vi "posctrl-drive-fwd-sim.vi"(11 "Motor Demand":dbl) -> (3 "Drive Speed Ft/Sec":dbl)   [LabVIEW 2019]
uses:
  <vilib>/Rock Robotics/WPI/ThirdParty/JAS_Junk/TrajLib/VI/TimeInterpDouble_New.vi
  <vilib>/Rock Robotics/WPI/ThirdParty/JAS_Junk/TrajLib/VI/TimeInterpDouble_AddSample.vi
  <vilib>/Rock Robotics/WPI/ThirdParty/JAS_Junk/TrajLib/VI/TimeInterpDouble_GetSample.vi
  <vilib>/Rock Robotics/WPI/ThirdParty/JAS_Junk/TrajLib/VI/TimeInterpDouble_SetMaxTime.vi
  <vilib>/Rock Robotics/WPI/ThirdParty/JAS_Junk/TrajLib/Util_GetTime.vi
  <vilib>/Rock Robotics/WPI/ThirdParty/JAS_Junk/TrajLib/LinearFilter_ResetToValue.vi
  <vilib>/Rock Robotics/WPI/ThirdParty/JAS_Junk/TrajLib/LinearFilter_Calculate.vi
  <vilib>/Rock Robotics/WPI/ThirdParty/JAS_Junk/TrajLib/VI/TimeInterpDouble_CleanUp.vi
  <vilib>/Rock Robotics/WPI/ThirdParty/JAS_Junk/TrajLib/MathUtil_Interpolate.vi
  <vilib>/Rock Robotics/WPI/ThirdParty/JAS_Junk/TrajLib/VI/Util_GetTime_U32.vi
  <vilib>/Rock Robotics/WPI/ThirdParty/JAS_Junk/TrajLib/VI/Util_GetTime_U64.vi
  <vilib>/gmath/interp.llb/Search Ordered Table.vi
  <vilib>/Rock Robotics/WPI/ThirdParty/JAS_Junk/TrajLib/LinearFilter_MovingAverage.vi
  <vilib>/Rock Robotics/WPI/ThirdParty/JAS_Junk/TrajLib/LinearFilter_LowPassBW1.vi
  <vilib>/Rock Robotics/WPI/ThirdParty/JAS_Junk/TrajLib/LinearFilter_LowPassBW2.vi
  <vilib>/Rock Robotics/WPI/ThirdParty/JAS_Junk/TrajLib/LinearFilter_HighPassBW1.vi
  <vilib>/Rock Robotics/WPI/ThirdParty/JAS_Junk/TrajLib/LinearFilter_HighPassBW2.vi
  <vilib>/Rock Robotics/WPI/ThirdParty/JAS_Junk/TrajLib/Trajectory_Library.lvlib
  <vilib>/ptbypt/NI_PtbyPt.lvlib
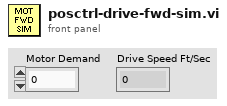
[diagram p1: front panel]
types:
  T1 = enum16{"Moving Average", "Low Pass 1st Order Butterworth", "Low Pass 2nd Order Butterworth", "High Pass 1st Order Butterworth", "High Pass 2nd Order Butterworth"}
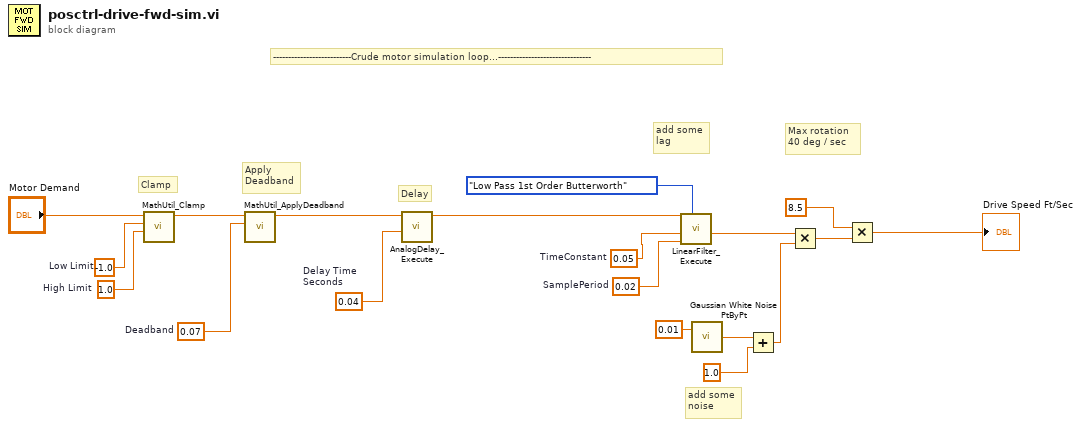
[diagram p0: block diagram]
diagram:
  w3 = 0.07  # Deadband
  w5 = 0.04  # Delay Time Seconds
  w9 = 1.0  # High Limit
  w8 = -1.0  # Low Limit
  w6 = 0.02  # SamplePeriod
  w19 = 0.05  # TimeConstant
  # "Apply\nDeadband"
  # "Delay"
  # "Max rotation \n40 deg / sec"
  # "Clamp"
  # "add some\nnoise"
  # "add some\nlag"
  # "--------------------------Crude motor simulation loop...-------------------------------"
  n1 = call <vilib>:"MathUtil_Clamp.vi"("High Limit"=w9, "Low Limit"=w8, "Value"="Motor Demand") -> ("Result"=w2:dbl)  [unwired: 8 in]
  n2 = call <vilib>:"MathUtil_ApplyDeadband.vi"("Deadband"=w3, "Value"=w2) -> ("Result"=w1:dbl)  [unwired: 9 in]
  n3 = call <vilib>:"AnalogDelay_Execute.vi"("Delay Time"=w5, "Input"=w1) -> ("Output"=w4:dbl)  [unwired: 8 in, 1 out]
  n4 = call <vilib>:"LinearFilter_Execute.vi"("Filter Type"=T1."Low Pass 1st Order Butterworth", "SamplePeriod"=w6, "TimeConstant"=w19, "Input"=w4) -> ("Output"=w13:dbl)  [unwired: 6 in, 1 out]
  n5 = call <vilib>:"Gaussian White Noise PtByPt.vi"("standard deviation"=0.01) -> ("Gaussian white noise"=w14:dbl)  [unwired: 2 in]
  n6 = Add(x=w14, y=1.0) -> (x+y=w12:dbl)
  n7 = Multiply(x=w13, y=w12) -> (x*y=w11:dbl)
  n8 = Multiply(x=8.5 ("value"), y=w11) -> (x*y=→"Drive Speed Ft/Sec":dbl)
